vi "Main.vi"() -> ()   [LabVIEW 2018, in "LGP5 Acquisition.lvlib"]
doc: "This template is based off of the Queued Message Handler design pattern and the Queued Message Handler project template that ships with LabVIEW.\n\nThe main difference is that the queue is private to this module and communication between modules is performed via Broadcast and Request events.\n\nRequest events are wrapped in public API methods and are handled in the Event Handling Loop (EHL) of this VI. Any module can register for Broadcast events sent by this module. The EHL generates messages based on user interface actions.\n\nThe Message Handling Loop (MHL) processes messages generated by the EHL, or by other messages. The messages are string values, so new messages can be added easily to the Message Cases case structure in the MHL. Each message cluster can also provide an optional value for Message Data, which is a variant that can be converted to whatever message-specific data is required.\n_____\nBased on Delacor QMH Project Template 4.1.0.59."
uses:
  LGP5 Acquisition.lvlib
  Module Data--cluster.ctl
  <vilib>/Delacor/Delacor QMH/Libraries/Message Queue_class/Delacor_lib_QMH_Message Queue.lvclass
  <vilib>/Delacor/Delacor QMH/Libraries/Message Queue_class/Delacor_lib_QMH_Enqueue Message (Single).vi
  <vilib>/ErrorRing/Error Ring.xnode
  <vilib>/Utility/error.llb/Error Cluster From Error Code.vi
  Clone Registration/Clone Registration.lvlib
  <vilib>/Delacor/Delacor QMH/Libraries/Cloneable Module Admin_class/Delacor_lib_QMH_Cloneable Module Admin.lvclass
  Stop Argument--cluster.ctl
  <vilib>/Utility/miscctls.llb/LVPointTypeDef.ctl
  Start Acquiring (Reply Payload)--cluster.ctl
  Start Acquiring Argument--cluster.ctl
panel:
  in  "Simulate MHL Error":bool
  in  "Simulate EHL Error":bool
  out "error out":errorcluster
  in  "Module Admin":refnum<class "Delacor_lib_QMH_Cloneable Module Admin.lvclass">
  out "Status":string
  # "Other QMH Modules communicate with this Module via its Public API (wrappers for its Request Events).\n\nThis Module communicates with other Modules via its Broadcast Events.\nAny module that wants to get these messages, just registers for this module's Broadcast events."
  # "This template is for the Delacor Modified Queued Message Handler design pattern.\n\nSee the block diagram for more information on how to use this template."
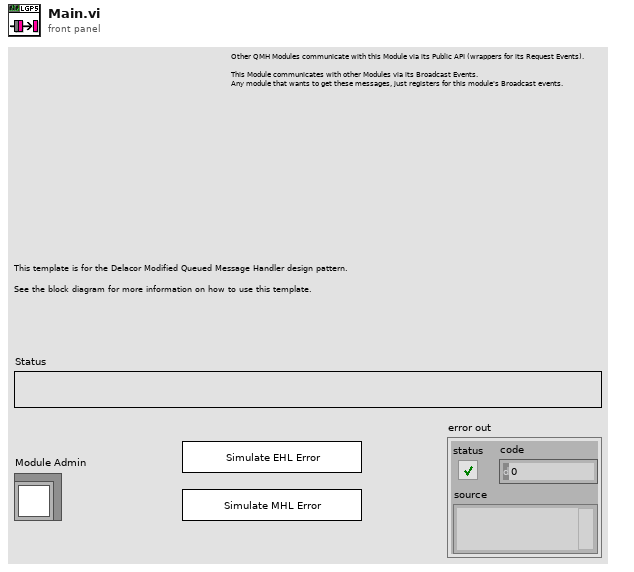
[diagram p1: front panel]
types:
  T1 = typedef "LGP5 Acquisition.lvlib/Request Events--cluster.ctl" = cluster{"Stop Module":refnum<user-event>, "Show Panel":refnum<user-event>, "Hide Panel":refnum<user-event>, "Show Diagram":refnum<user-event>, "Get Module Execution Status":refnum<user-event>, "Start Acquiring":refnum<user-event>}
  T2 = typedef "LGP5 Acquisition.lvlib/Module Data--cluster.ctl" = cluster{"Status":string}
  T3 = enum32{"invalid lock state", "Not Locked", "Locked (No Password)", "Password-protected"}
  T4 = typedef "LGP5 Acquisition.lvlib/Stop Argument--cluster.ctl" = cluster{"Module ID":i32, "Origin":string, "Exit via Stop Module Req?":bool, "Wait for Module to stop?":bool}
  T5 = typedef "LGP5 Acquisition.lvlib/Start Acquiring Argument--cluster.ctl" = cluster{"Module ID":i32, "Wait Notifier":refnum<notifier>, "wait for reply":bool}
  T6 = typedef "LVPointTypeDef.ctl" = cluster{"Horizontal":i16, "Vertical":i16}
  T7 = enum32{"Invalid", "Standard", "Closed", "Hidden", "Minimized", "Maximized"}
  T8 = typedef "LGP5 Acquisition.lvlib/Start Acquiring (Reply Payload)--cluster.ctl" = cluster{"HW ID":string, "Start Acquiring_error":errorcluster}
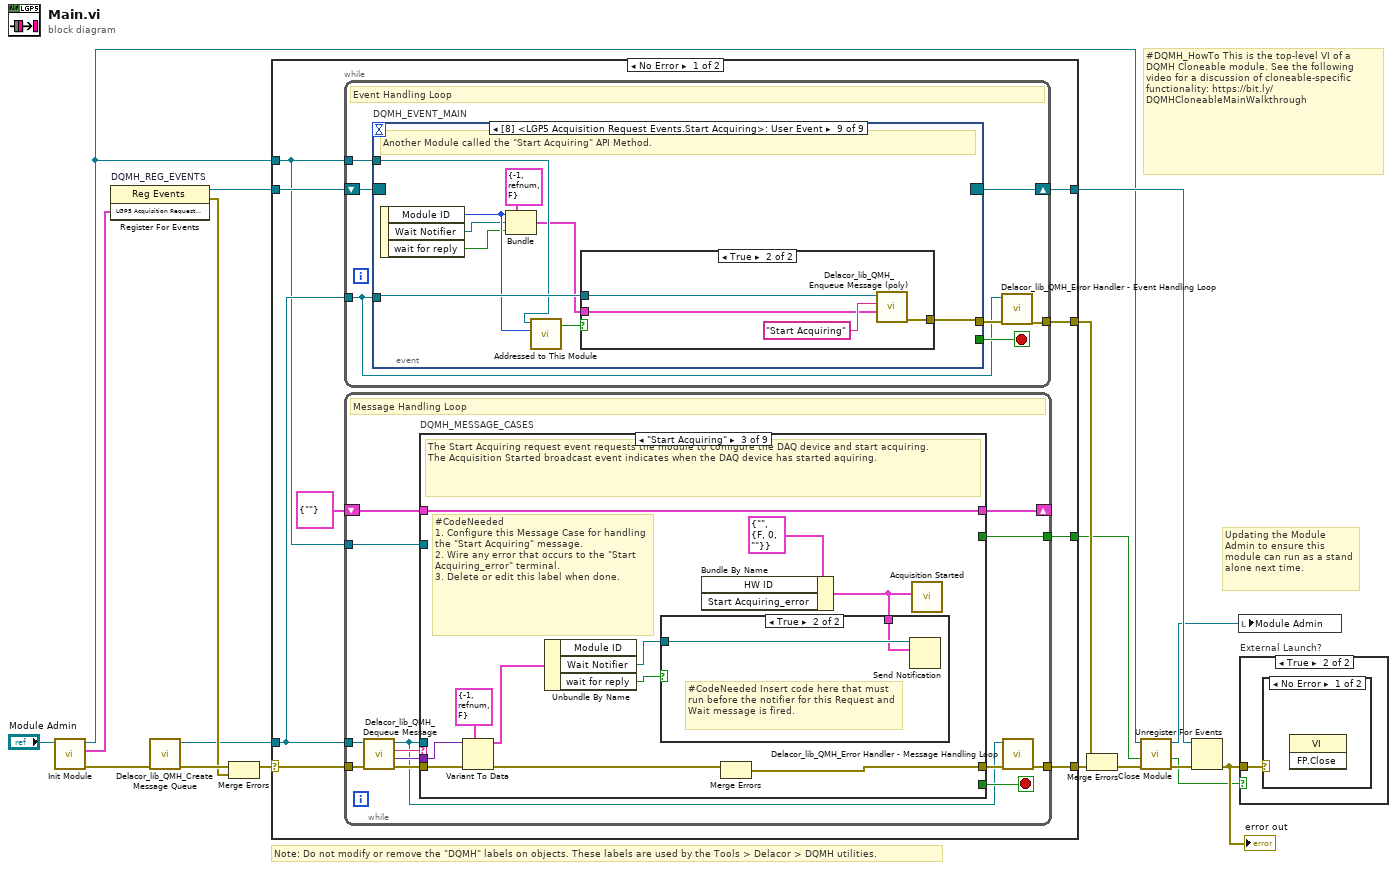
[diagram p0: block diagram]
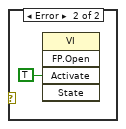
[diagram p3: hidden frame]
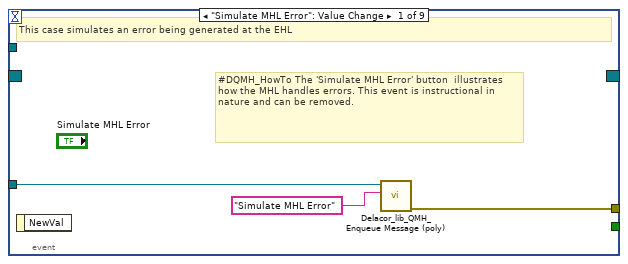
[diagram p4: hidden frame]
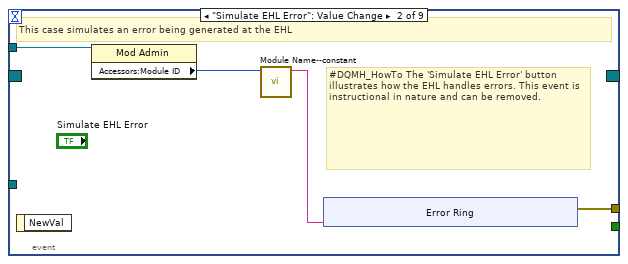
[diagram p5: hidden frame]
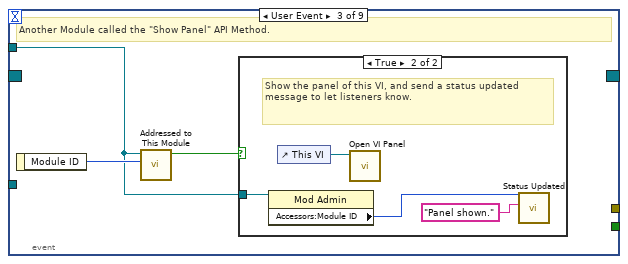
[diagram p6: hidden frame]
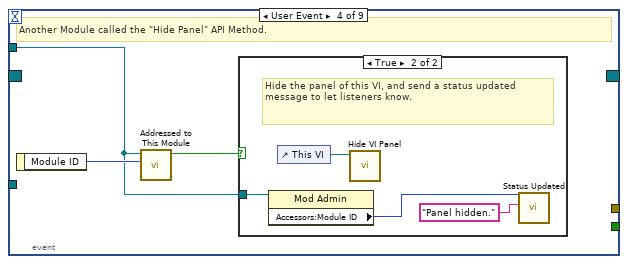
[diagram p8: hidden frame]
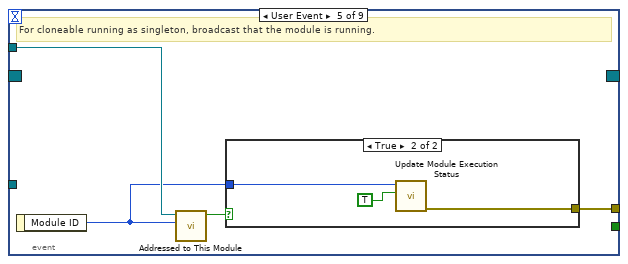
[diagram p10: hidden frame]
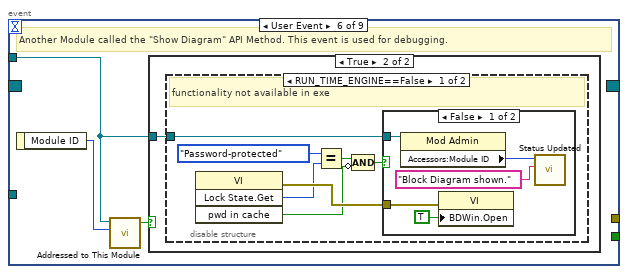
[diagram p12: hidden frame]
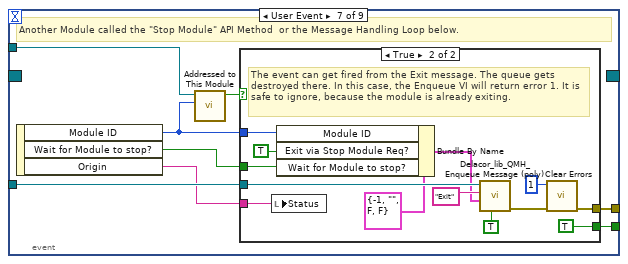
[diagram p16: hidden frame]
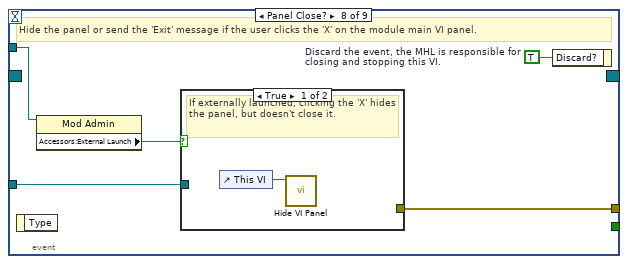
[diagram p18: hidden frame]
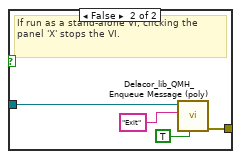
[diagram p19: hidden frame]
diagram:
  # "#DQMH_HowTo This is the top-level VI of a DQMH Cloneable module. See the following video for a discussion of cloneable-specific functionality: https://bit.ly/DQMHCloneableMainWalkthrough"
  # "Note: Do not modify or remove the \"DQMH\" labels on objects. These labels are used by the Tools > Delacor > DQMH utilities."
  # "Updating the Module Admin to ensure this module can run as a stand alone next time."
  n1 = call "Init Module.vi"("Cloneable Module Admin in"="Module Admin") -> ("error out"=w15:errorcluster, "LGP5 Acquisition Request Events"=w7:T1, "Cloneable Module Admin out"=w4:refnum<class "Delacor_lib_QMH_Cloneable Module Admin.lvclass">)  [unwired: 8 in]
  n2 = register-events "DQMH_REG_EVENTS"(w7) -> (reference out=w8:refnum<event-registration>, error out=w10:errorcluster)  [unwired: 2 in]
  n3 = call <vilib>:"Delacor_lib_QMH_Create Message Queue.vi"("error in (no error)"=w15) -> ("error out"=w12:errorcluster, "Message Queue"=w6:refnum<class "Delacor_lib_QMH_Message Queue.lvclass">)  [unwired: 9 in]
  n4 = Merge Errors(w12, w10) -> (w11:errorcluster)
  n5 = case shown="No Error" w11 {
    selector: w11 -> [w25 w254]
    tunnel: [w27 w254] -> w16
    tunnel: [w24 w253] -> w9
    tunnel: w8 -> [w22 w253]
    tunnel: w6 -> [w21 _]
    tunnel: [w26 _] -> w17
    tunnel: w4 -> [w20 w249]
    tunnel: [w19 _] -> w2
    frame No Error {
      n6 = while {
        tunnel: w21 -> [w28]
        shift-right: [w31] -> w24
        shift-left: w22 -> [w32]
        tunnel: [w33] -> w26
        tunnel: w20 -> [w29]
        stop <- w30 stop-if-true
        # "Event Handling Loop"
        n7 = event "DQMH_EVENT_MAIN" shown="[8] <LGP5 Acquisition Request Events.Start Acquiring>: User Event" {
          selector: w32 -> [_ _ _ _ _ _ _ _ _]
          dyn-events: [_ _ _ _ _ _ _ _ _] -> w31
          timeout: _ -> [_ _ _ _ _ _ _ _ _]
          tunnel: [_ _ _ _ _ _ w89 _ _] -> w30
          tunnel: w28 -> [w36 _ _ _ _ _ w92 w108 w125]
          tunnel: [w37 w41 _ _ w66 _ w93 w111 w117] -> w34
          tunnel: w29 -> [_ w40 w49 w56 w64 w70 w91 w109 w123]
          event "Simulate MHL Error": Value Change {
            # "#DQMH_HowTo The 'Simulate MHL Error' button  illustrates how the MHL handles errors. This event is instructional in nature and can be removed."
            # "This case simulates an error being generated at the EHL"
            n8 = event-data() -> ()  [unwired: 1 in, 1 out]
            n9 = call-poly <vilib>:"Delacor_lib_QMH_Enqueue Message (poly).vi"("Message"="Simulate MHL Error", "Message Queue in"=w36) -> ("error out"=w37:errorcluster)  [unwired: 8 in, 1 out]
          }
          event "Simulate EHL Error": Value Change {
            # "#DQMH_HowTo The 'Simulate EHL Error' button  illustrates how the EHL handles errors. This event is instructional in nature and can be removed."
            # "This case simulates an error being generated at the EHL"
            n10 = event-data() -> ()  [unwired: 1 in, 1 out]
            n11 = property class="Mod Admin"(reference=w40) -> ("Accessors:Module ID"=w39:i32)  [unwired: 1 in, 2 out]
            n12 = call "Module Name--constant.vi"("Module ID"=w39) -> ("Module Name"=w38:string)  [unwired: 10 in]
            n13 = xnode "Error Ring"("parameter 0"=w38) -> ("error out"=w41:errorcluster)
          }
          event User Event {
            # "Another Module called the \"Show Panel\" API Method."
            n14 = event-data() -> ("Module ID"=w50:i32)  [unwired: 1 in]
            n15 = call "Addressed to This Module.vi"("Module ID from Argument"=w50, "Module Admin"=w49) -> ("Addressed to this instance?"=w51:bool)  [unwired: 8 in, 1 out]
            n16 = case shown="True" w51 {
              tunnel: w49 -> [_ w53]
              frame False {
              }
              frame True {
                # "Show the panel of this VI, and send a status updated message to let listeners know."
                n17 = property class="Mod Admin"(reference=w53) -> ("Accessors:Module ID"=w52:i32)  [unwired: 1 in, 2 out]
                n18 = control-ref of="This VI"() -> (w55:refnum<vi>)
                n19 = call "Open VI Panel.vi"("VI"=w55) -> ()  [unwired: 10 in, 1 out]
                n20 = call "Status Updated.vi"("Status"="Panel shown." ("format string"), "Module ID"=w52) -> ()  [unwired: 9 in, 1 out]
              }
            }
          }
          event User Event {
            # "Another Module called the \"Hide Panel\" API Method."
            n21 = event-data() -> ("Module ID"=w57:i32)  [unwired: 1 in]
            n22 = call "Addressed to This Module.vi"("Module ID from Argument"=w57, "Module Admin"=w56) -> ("Addressed to this instance?"=w58:bool)  [unwired: 8 in, 1 out]
            n23 = case shown="True" w58 {
              tunnel: w56 -> [_ w60]
              frame False {
              }
              frame True {
                # "Hide the panel of this VI, and send a status updated message to let listeners know."
                n24 = property class="Mod Admin"(reference=w60) -> ("Accessors:Module ID"=w59:i32)  [unwired: 1 in, 2 out]
                n25 = control-ref of="This VI"() -> (w62:refnum<vi>)
                n26 = call "Hide VI Panel.vi"("VI"=w62) -> ()  [unwired: 10 in, 1 out]
                n27 = call "Status Updated.vi"("Status"="Panel hidden." ("format string"), "Module ID"=w59) -> ()  [unwired: 9 in, 1 out]
              }
            }
          }
          event User Event {
            # "For cloneable running as singleton, broadcast that the module is running."
            n28 = event-data() -> ("Module ID"=w63:i32)  [unwired: 1 in]
            n29 = call "Addressed to This Module.vi"("Module ID from Argument"=w63, "Module Admin"=w64) -> ("Addressed to this instance?"=w65:bool)  [unwired: 8 in, 1 out]
            n30 = case shown="True" w65 {
              tunnel: [_ w69] -> w66
              tunnel: w63 -> [_ w68]
              frame False {
              }
              frame True {
                n31 = call "Update Module Execution Status.vi"("Running?"=TRUE, "Module ID"=w68) -> ("error out"=w69:errorcluster)  [unwired: 9 in]
              }
            }
          }
          event User Event {
            # "Another Module called the \"Show Diagram\" API Method. This event is used for debugging."
            n32 = event-data() -> ("Module ID"=w71:i32)  [unwired: 1 in]
            n33 = call "Addressed to This Module.vi"("Module ID from Argument"=w71, "Module Admin"=w70) -> ("Addressed to this instance?"=w72:bool)  [unwired: 8 in, 1 out]
            n34 = case shown="True" w72 {
              tunnel: w70 -> [_ w73]
              frame False {
              }
              frame True {
                n35 = disable-structure shown="RUN_TIME_ENGINE==False" {
                  disable-tunnel: w73 -> [w74 _]
                  frame condition #0 (active) {
                    # "functionality not available in exe"
                    n36 = invoke class="VI" method="Lock State.Get"() -> (error out=w80:errorcluster, "Get Lock State"=w79:T3, "pwd in cache"=w76:bool)  [unwired: 4 in, 1 out]
                    n37 = Equal?(x=T3."Password-protected", y=w79) -> (x = y?=w77:bool)
                    n38 = Compound Arithmetic op=AND(w77, invert w76) -> (w75:bool)
                    n39 = case shown="False" w75 {
                      tunnel: w80 -> [w85 _]
                      tunnel: w74 -> [w82 _]
                      frame False {
                        n40 = property class="Mod Admin"(reference=w82) -> ("Accessors:Module ID"=w81:i32)  [unwired: 1 in, 2 out]
                        n41 = property class="VI"(error in=w85, "BDWin.Open"=TRUE ("Block Diagram Window:Open")) -> ()  [unwired: 1 in, 2 out]
                        n42 = call "Status Updated.vi"("Status"="Block Diagram shown." ("format string"), "Module ID"=w81) -> ()  [unwired: 9 in, 1 out]
                      }
                      frame True {
                        # "Password-protected VI, and the password is not in the cache. Do not show the diagram."
                      }
                    }
                  }
                  frame condition #1 {
                  }
                }
              }
            }
          }
          event User Event {
            # "Another Module called the \"Stop Module\" API Method  or the Message Handling Loop below."
            n43 = event-data() -> ("Module ID"=w87:i32, "Wait for Module to stop?"=w88:bool, "Origin"=w86:string)  [unwired: 1 in]
            n44 = call "Addressed to This Module.vi"("Module ID from Argument"=w87, "Module Admin"=w91) -> ("Addressed to this instance?"=w90:bool)  [unwired: 8 in, 1 out]
            n45 = case shown="True" w90 {
              tunnel: [_ w105] -> w93
              tunnel: w92 -> [_ w101]
              tunnel: [_ TRUE] -> w89
              tunnel: w88 -> [_ w96]
              tunnel: w87 -> [_ w98]
              tunnel: w86 -> [_ w94]
              frame False {
              }
              frame True {
                # "The event can get fired from the Exit message. The queue gets destroyed there. In this case, the Enqueue VI will return error 1. It is safe to ignore, because the module is already exiting."
                n46 = local write "Status"(w94) -> ()
                n47 = Bundle By Name(cluster=T4 {"Module ID"=-1, "Origin"="", "Exit via Stop Module Req?"=FALSE, "Wait for Module to stop?"=FALSE} ("Stop Argument"), "Module ID"=w98, "Exit via Stop Module Req?"=TRUE, "Wait for Module to stop?"=w96) -> (w95:T4)
                n48 = call-poly <vilib>:"Delacor_lib_QMH_Enqueue Message (poly).vi"("Priority Message? (F)"=TRUE, "Message Data"=w95, "Message"="Exit", "Message Queue in"=w101) -> ("error out"=w106:errorcluster)  [unwired: 6 in, 1 out]
                n49 = call <vilib>:"Clear Errors.vi"("error in (no error)"=w106, "specific error code to clear (0: all)"=1) -> ("error out"=w105:errorcluster)  [unwired: 4 in, 1 out]
              }
            }
          }
          event Panel Close? {
            w110 = TRUE  # Discard the event, the MHL is responsible for closing and stopping this VI.
            # "Hide the panel or send the 'Exit' message if the user clicks the 'X' on the module main VI panel."
            n50 = event-data() -> ()  [unwired: 1 in, 1 out]
            n51 = property class="Mod Admin"(reference=w109) -> ("Accessors:External Launch"=w107:bool)  [unwired: 1 in, 2 out]
            n52 = case shown="True" w107 {
              tunnel: w108 -> [_ w115]
              tunnel: [_ w116] -> w111
              frame True {
                # "If externally launched, clicking the 'X' hides the panel, but doesn't close it."
                n53 = control-ref of="This VI"() -> (w112:refnum<vi>)
                n54 = call "Hide VI Panel.vi"("VI"=w112) -> ()  [unwired: 10 in, 1 out]
              }
              frame False {
                # "If run as a stand-alone VI, clicking the panel 'X' stops the VI."
                n55 = call-poly <vilib>:"Delacor_lib_QMH_Enqueue Message (poly).vi"("Priority Message? (F)"=TRUE, "Message"="Exit", "Message Queue in"=w115) -> ("error out"=w116:errorcluster)  [unwired: 7 in, 1 out]
              }
            }
            n56 = event-data("Discard?"=w110) -> ()  [unwired: 1 in, 1 out]
          }
          event User Event {
            # "Another Module called the \"Start Acquiring\" API Method."
            n57 = event-data() -> ("Module ID"=w120:i32, "Wait Notifier"=w119:refnum<notifier>, "wait for reply"=w118:bool)  [unwired: 1 in]
            n58 = Bundle(cluster=T5 {"Module ID"=-1, "Wait Notifier"=refnum, "wait for reply"=FALSE} ("Start Acquiring Argument"), "Module ID"=w120, "Wait Notifier"=w119, "wait for reply"=w118) -> (w121:T5)
            n59 = call "Addressed to This Module.vi"("Module ID from Argument"=w120, "Module Admin"=w123) -> ("Addressed to this instance?"=w124:bool)  [unwired: 8 in, 1 out]
            n60 = case shown="True" w124 {
              tunnel: w125 -> [_ w129]
              tunnel: w121 -> [_ w127]
              tunnel: [_ w126] -> w117
              frame False {
              }
              frame True {
                n61 = call-poly <vilib>:"Delacor_lib_QMH_Enqueue Message (poly).vi"("Message Data"=w127, "Message"="Start Acquiring", "Message Queue in"=w129) -> ("error out"=w126:errorcluster)  [unwired: 7 in, 1 out]
              }
            }
          }
        }
        n62 = call-dynamic "Delacor_lib_QMH_Error Handler - Event Handling Loop.vi"("error in (no error)"=w34, "Message Queue in"=w28) -> ("dup error in"=w33:errorcluster)  [unwired: 8 in, 1 out]
      }
      n63 = while {
        tunnel: w21 -> [w133]
        shift-right: [w137] -> _
        shift-left: T2 {"Status"=""} ("Data Cluster") -> [w138]
        tunnel: w25 -> [w141]
        tunnel: [w139] -> w27
        tunnel: w20 -> [w131]
        tunnel: [w130] -> w19
        stop <- w136 stop-if-true
        # "Message Handling Loop"
        n64 = call-dynamic "Delacor_lib_QMH_Dequeue Message.vi"("error in (no error)"=w141, "Message Queue in"=w133) -> ("error out"=w140:errorcluster, "Message Data"=w134:variant, "Message"=w135:string, "Message Queue out"=w132:refnum<class "Delacor_lib_QMH_Message Queue.lvclass">)  [unwired: 6 in]
        n65 = case "DQMH_MESSAGE_CASES" shown="\"Start Acquiring\"" w135 {
          selector: w135 -> [_ _ _ _ _ _ _ _ w234]
          tunnel: w132 -> [_ _ _ _ _ w184 _ w224 _]
          tunnel: w140 -> [w161 w165 w176 w181 w183 w194 w207 w230 w236]
          tunnel: [w159 w165 w166 w180 w183 w190 w206 w227 w237] -> w142
          tunnel: w138 -> [w152 w164 w175 w179 w182 w189 w204 w223 w235]
          tunnel: [w151 w164 w175 w179 w182 w189 w204 w223 w235] -> w137
          tunnel: [_ _ _ _ _ _ _ w222 _] -> w136
          tunnel: w134 -> [_ _ w173 _ _ w188 _ w220 _]
          tunnel: w131 -> [w146 _ _ _ _ w187 w202 w216 w232]
          tunnel: [_ _ _ _ _ _ _ w218 _] -> w130
          frame "Initialize" {
            w143 = "Initial Message" ("Initial Message")
            # "#CodeNeeded - Initialize the appearance of the front panel."
            # "#CodeNeeded - Initialize your state data here."
            # "Initialize - Any operation that needs to be done before the module can receive messages. Synchronize Caller Events.vi will inform Start Module.vi that the module has launched and is ready to receive messages. Module Did Init.vi will broadcast that the module initialized."
            n66 = call "Synchronize Caller Events.vi"("error in (no error)"=w161, "Module Admin"=w146) -> ("error out"=w160:errorcluster, "Module Admin out"=w145:refnum<class "Delacor_lib_QMH_Cloneable Module Admin.lvclass">)  [unwired: 8 in]
            n67 = property class="Mod Admin"(reference=w145) -> ("Accessors:Module ID"=w148:i32, "Accessors:External Launch"=w147:bool)  [unwired: 1 in, 2 out]
            n68 = call "Module Name--constant.vi"("Module ID"=w148) -> ("Module Name"=w156:string)  [unwired: 10 in]
            n69 = property class="VI"("Front Panel.Title"=w156) -> (reference out=w158:refnum<vi>, error out=w163:errorcluster)  [unwired: 2 in]
            n70 = Select(t=T7."Hidden" ("State"), s=w147, f=T7."Standard" ("State")) -> (s? t:f=w153:T7)
            n71 = invoke class="VI" method="FP.Open"(reference=w158, error in=w163, "State"=w153) -> (reference out=w157:refnum<vi>, error out=w162:errorcluster)  [unwired: 2 in, 3 out]
            n72 = call "Module Name--constant.vi"("Module ID"=w148) -> ("Module Name"=w149:string)  [unwired: 10 in]
            n73 = Bundle By Name(cluster=w152, "Status"=w143) -> (w151:T2)
            n74 = invoke class="VI" method="FP.Center"(reference=w157, error in=w162) -> ()  [unwired: 1 in, 3 out]
            n75 = property on="Pane" class="Pane"("Origin"=T6 {"Horizontal"=0, "Vertical"=0}) -> ()  [unwired: 2 in, 2 out]
            n76 = call "Module Did Init.vi"("error in (no error)"=w160, "Initialized?"=TRUE, "Origin"=w149, "Module ID"=w148) -> ("error out"=w159:errorcluster)  [unwired: 7 in]
            "Status" <- w143
          }
          frame "--- Module Specific ---" {
            # "Separator -- The following cases handle messages specific to this Module."
          }
          frame "Start Acquiring" {
            # "#CodeNeeded\n1. Configure this Message Case for handling the \"Start Acquiring\" message.\n2. Wire any error that occurs to the \"Start Acquiring_error\" terminal.\n3. Delete or edit this label when done."
            # "The Start Acquiring request event requests the module to configure the DAQ device and start acquiring.\nThe Acquisition Started broadcast event indicates when the DAQ device has started aquiring."
            n77 = Variant To Data(error in=w176, type=T5 {"Module ID"=-1, "Wait Notifier"=refnum, "wait for reply"=FALSE} ("Start Acquiring Argument"), Variant=w173) -> (data=w171:T5, error out=w174:errorcluster)
            n78 = Unbundle By Name(w171) -> ("Wait Notifier"=w170:refnum<notifier>, "wait for reply"=w169:bool)  [unwired: 1 out]
            n79 = Bundle By Name(cluster=T8 {"HW ID"="", "Start Acquiring_error"={"status"=FALSE, "code"=0, "source"=""}} ("Start Acquiring (Reply Payload)")) -> (w168:T8)  [unwired: 2 in]
            n80 = case shown="True" w169 {
              tunnel: w170 -> [_ w178]
              tunnel: w168 -> [_ w177]
              frame False {
              }
              frame True {
                # "#CodeNeeded Insert code here that must run before the notifier for this Request and Wait message is fired."
                n81 = Send Notification(notification=w177, notifier=w178) -> ()  [unwired: 1 in, 2 out]
              }
            }
            n82 = Merge Errors(w174) -> (w166:errorcluster)  [unwired: 1 in]
            n83 = call "Acquisition Started.vi"("Reply Payload"=w168) -> ()  [unwired: 10 in, 1 out]
          }
          frame "---Copy This Frame---" {
            # "Duplicate this frame when creating new messages.  Change this comment in the duplicated frame to describe this message."
            n84 = Merge Errors(w181) -> (w180:errorcluster)
          }
          frame "--- Exit and Error Handling---" {
            # "Separator - the following cases handle errors and exit messages."
          }
          frame "Error" {
            # "#CodeRecommended - If you ever change the name of this \"Error\" message, you'll need to update the name in the Check Loop Error.vi as well."
            # "#CodeRecommended - If the module is running in standalone mode (External Launch = FALSE), this code will pop up an error dialog and call the 'Exit' message if an error occurs. Add more fine-grained error handling here."
            # "Error - Check the error message data and respond accordingly. This message is sent by the \"Error Handler\" VIs at the end of each loop in this application."
            n85 = property class="Mod Admin"(reference=w187) -> ("Accessors:External Launch"=w185:bool, "Accessors:Module ID"=w186:i32)  [unwired: 1 in, 2 out]
            n86 = Variant To Data(error in=w194, type=errorcluster {"status"=FALSE, "code"=0, "source"=""} ("error constant"), Variant=w188) -> (data=w195:errorcluster, error out=w192:errorcluster)
            n87 = call "Error Reported.vi"("Error"=w195, "Module ID"=w186) -> ()  [unwired: 9 in, 1 out]
            n88 = case shown="False" w185 {
              tunnel: [w200 _] -> w191
              tunnel: w184 -> [w198 _]
              tunnel: w195 -> [w199 _]
              frame False {
                # "If the module is running standalone, then pop up an error dialog and call the \"Exit\" message."
                n89 = call <vilib>:"Simple Error Handler.vi"("error in (no error)"=w199) -> ()  [unwired: 4 in, 5 out]
                n90 = call-poly <vilib>:"Delacor_lib_QMH_Enqueue Message (poly).vi"("Priority Message? (F)"=TRUE, "Message"="Exit", "Message Queue in"=w198) -> ("error out"=w200:errorcluster)  [unwired: 7 in, 1 out]
              }
              frame True {
                # "If the module was launched externally, calling the Error Reported broadcast VI is the only action performed by the \"Error\" message. The module's caller can then process the error appropriately."
              }
            }
            n91 = Merge Errors(w192, w191) -> (w190:errorcluster)
            n92 = local write "error out"(w190) -> ()
          }
          frame "Simulate MHL Error" {
            # "#DQMH_HowTo The 'Simulate MHL Error' button  illustrates how the MHL handles errors. This event is instructional in nature and can be removed."
            # "Simulate an error occurring at the MHL"
            n93 = property class="Mod Admin"(reference=w202) -> ("Accessors:Module ID"=w203:i32)  [unwired: 1 in, 2 out]
            n94 = call "Module Name--constant.vi"("Module ID"=w203) -> ("Module Name"=w201:string)  [unwired: 10 in]
            n95 = xnode "Error Ring"("parameter 0"=w201) -> ("error out"=w205:errorcluster)
            n96 = Merge Errors(w207, w205) -> (w206:errorcluster)
          }
          frame "Exit" {
            w221 = 91  # 91: not all Exit messages will have an argument
            w222 = TRUE  # Stop the VI
            # "Release the message queue reference"
            # "#CodeNeeded - Add any required cleanup code here."
            # "Exit - Exit the application."
            n97 = Variant To Data(error in=w230, type=T4 {"Module ID"=-1, "Origin"="", "Exit via Stop Module Req?"=FALSE, "Wait for Module to stop?"=FALSE} ("Stop Argument"), Variant=w220) -> (data=w217:T4, error out=w225:errorcluster)
            n98 = call <vilib>:"Clear Errors.vi"("error in (no error)"=w225, "specific error code to clear (0: all)"=w221) -> ("error out"=w229:errorcluster)  [unwired: 4 in, 1 out]
            n99 = control-ref of="This VI"() -> (w215:refnum<vi>)
            n100 = call-dynamic "Delacor_lib_QMH_Release Message Queue.vi"("error in (no error)"=w229, "Message Queue"=w224) -> ("error out"=w228:errorcluster)  [unwired: 9 in]
            n101 = call "Handle Exit.vi"("Stop Argument"=w217, "Module Admin in"=w216, "VI reference"=w215) -> ("error out"=w226:errorcluster, "Wait for Stop?"=w218:bool)  [unwired: 7 in]
            n102 = Merge Errors(w228, w226) -> (w227:errorcluster)
          }
          frame Default {
            # "'Default' case only runs if there is a message that isn't defined in any of the other cases.  Output a programming error."
            n103 = property class="Mod Admin"(reference=w232) -> ("Accessors:Module ID"=w231:i32)  [unwired: 1 in, 2 out]
            n104 = call "Module Name--constant.vi"("Module ID"=w231) -> ("Module Name"=w233:string)  [unwired: 10 in]
            n105 = xnode "Error Ring"("parameter 0"=w234, "parameter 1"=w233) -> ("error out"=w238:errorcluster)
            n106 = Merge Errors(w236, w238) -> (w237:errorcluster)
          }
        }
        n107 = call-dynamic "Delacor_lib_QMH_Error Handler - Message Handling Loop.vi"("error in (no error)"=w142, "Message Queue in"=w132) -> ("dup error in"=w139:errorcluster)  [unwired: 8 in, 1 out]
      }
    }
    frame Error {
      n108 = call "Synchronize Caller Events.vi"("Module Admin"=w249) -> ("Module Admin out"=w248:refnum<class "Delacor_lib_QMH_Cloneable Module Admin.lvclass">)  [unwired: 9 in, 1 out]
      n109 = property class="Mod Admin"(reference=w248) -> ("Accessors:Module ID"=w247:i32)  [unwired: 1 in, 2 out]
      n110 = call "Module Name--constant.vi"("Module ID"=w247) -> ("Module Name"=w252:string)  [unwired: 10 in]
      n111 = call "Remove.vi"("Module ID"=w247) -> ()  [unwired: 9 in, 2 out]
      n112 = Format Into String(format string="An error occurred during initialization. %s is no longer running.", w252) -> (resulting string=w250:string)  [unwired: 2 in, 1 out]
      n113 = call "Error Reported.vi"("Additional Information"=w250, "Error"=w254, "Module ID"=w247) -> ()  [unwired: 8 in, 1 out]
    }
  }
  n114 = Merge Errors(w17, w16) -> (w18:errorcluster)
  n115 = call "Close Module.vi"("error in (no error)"=w18, "Wait for stop?"=w2, "Module Admin in"=w4) -> ("error out"=w14:errorcluster, "External Launch"=w1:bool, "Module Admin out"=w3:refnum<class "Delacor_lib_QMH_Cloneable Module Admin.lvclass">)  [unwired: 6 in]
  n116 = Unregister For Events(event registration refnum=w9, error in=w14) -> (error out=w13:errorcluster)
  "error out" <- w13
  n117 = local write "Module Admin"(w3) -> ()
  n118 = case "External Launch?" shown="True" w1 {
    tunnel: w13 -> [_ w255]
    frame False {
    }
    frame True {
      n119 = case shown="No Error" w255 {
        frame No Error {
          n120 = invoke class="VI" method="FP.Close"() -> ()  [unwired: 3 in, 3 out]
        }
        frame Error {
          n121 = invoke class="VI" method="FP.Open"("Activate"=TRUE ("Activate?")) -> ()  [unwired: 4 in, 5 out]
        }
      }
    }
  }
